vi "Grafici MANAGER REPORT.vi"() -> ()   [LabVIEW 2019]
uses:
  Global percorso impostazioni.vi
  TypeDef/Definizione_plot.ctl
  TypeDef/Definizione_Grafico_REPORT_OLD.ctl
panel:
  out "deleted portion":T1[](array[typedef]) {"PLOT"."GRANDEZZA Y" items=["Banco", "Anno", "Numero", "N° tabella", "Misura", "Tipo prova", "Progressivo Acq", "tempo[h:m:s]", "tempo acq[min]", "f [Hz]", "Uav [V]", "Iav [A]", "Tq [Nm]", "n [rpm]", "P1 [kW]", "P1 n[kW]", "Q [m3/h]", "Q n[m3/h]", "Q [l/min]", "Q n[l/min]", "H1 [m]", "Dislivello [m]", "Hdinamica [m]", "HvAsp [m]", "HvMand [m]", "HvTot [m]", "H2 [m]", "Htot [m]", "Htot n[m]", "P3 (Phyd) [kW]", "P3 (Phyd) n[kW]", "P2 [kW]", "P2 n[kW]", "P2 n ps[kW]", "eta motore [%]", "eta pompa [%]", "eta pompa n[%]", "eta gruppo [%]", "eta gruppo n[%]", "T acqua [°C]", "Densità liquido [kg/m3]", "P barometrica [mbar]", "pf", "Uch1 [V]", "Uch2 [V]", "Uch3 [V]", "Ich1 [A]", "Ich2 [A]", "Ich3 [A]", "Temp.amb[°C]", "Ru-w [ohm]", "DTavvolg. [°C]", "Tamb Freddo [°C]", "Ru-w Freddo [ohm]", "Tc1[°C]", "Tc2[°C]", "Tc3[°C]", "Tc4[°C]", "Tc5", "Tc6", "Tc7", "Tc8", "H1[Bar]", "H2[bar]", "P premist.[Bar]", "Pserb[bar]", "n°NPSH", "NPSH", "Htot Ref[m]", "NPSH_%caduta", "%caduta", "Qref [m3/h]", "MEI"]; "PLOT"."GRANDEZZA X" items=["Banco", "Anno", "Numero", "N° tabella", "Misura", "Tipo prova", "Progressivo Acq", "tempo[h:m:s]", "tempo acq[min]", "f [Hz]", "Uav [V]", "Iav [A]", "Tq [Nm]", "n [rpm]", "P1 [kW]", "P1 n[kW]", "Q [m3/h]", "Q n[m3/h]", "Q [l/min]", "Q n[l/min]", "H1 [m]", "Dislivello [m]", "Hdinamica [m]", "HvAsp [m]", "HvMand [m]", "HvTot [m]", "H2 [m]", "Htot [m]", "Htot n[m]", "P3 (Phyd) [kW]", "P3 (Phyd) n[kW]", "P2 [kW]", "P2 n[kW]", "P2 n ps[kW]", "eta motore [%]", "eta pompa [%]", "eta pompa n[%]", "eta gruppo [%]", "eta gruppo n[%]", "T acqua [°C]", "Densità liquido [kg/m3]", "P barometrica [mbar]", "pf", "Uch1 [V]", "Uch2 [V]", "Uch3 [V]", "Ich1 [A]", "Ich2 [A]", "Ich3 [A]", "Temp.amb[°C]", "Ru-w [ohm]", "DTavvolg. [°C]", "Tamb Freddo [°C]", "Ru-w Freddo [ohm]", "Tc1[°C]", "Tc2[°C]", "Tc3[°C]", "Tc4[°C]", "Tc5", "Tc6", "Tc7", "Tc8", "H1[Bar]", "H2[bar]", "P premist.[Bar]", "Pserb[bar]", "n°NPSH", "NPSH", "Htot Ref[m]", "NPSH_%caduta", "%caduta", "Qref [m3/h]", "MEI"]; "Assi grafico"."ASSE X" items=["X 1", "X 2"]; "Assi grafico"."ASSE Y" items=["Y 1", "Y 2", "Y 3", "Y 4"]}
  out "Array plot":T1[](array[typedef]) {"PLOT"."GRANDEZZA Y" items=["Banco", "Anno", "Numero", "N° tabella", "Misura", "Tipo prova", "Progressivo Acq", "tempo[h:m:s]", "tempo acq[min]", "f [Hz]", "Uav [V]", "Iav [A]", "Tq [Nm]", "n [rpm]", "P1 [kW]", "P1 n[kW]", "Q [m3/h]", "Q n[m3/h]", "Q [l/min]", "Q n[l/min]", "H1 [m]", "Dislivello [m]", "Hdinamica [m]", "HvAsp [m]", "HvMand [m]", "HvTot [m]", "H2 [m]", "Htot [m]", "Htot n[m]", "P3 (Phyd) [kW]", "P3 (Phyd) n[kW]", "P2 [kW]", "P2 n[kW]", "P2 n ps[kW]", "eta motore [%]", "eta pompa [%]", "eta pompa n[%]", "eta gruppo [%]", "eta gruppo n[%]", "T acqua [°C]", "Densità liquido [kg/m3]", "P barometrica [mbar]", "pf", "Uch1 [V]", "Uch2 [V]", "Uch3 [V]", "Ich1 [A]", "Ich2 [A]", "Ich3 [A]", "Temp.amb[°C]", "Ru-w [ohm]", "DTavvolg. [°C]", "Tamb Freddo [°C]", "Ru-w Freddo [ohm]", "Tc1[°C]", "Tc2[°C]", "Tc3[°C]", "Tc4[°C]", "Tc5", "Tc6", "Tc7", "Tc8", "H1[Bar]", "H2[bar]", "P premist.[Bar]", "Pserb[bar]", "n°NPSH", "NPSH", "Htot Ref[m]", "NPSH_%caduta", "%caduta", "Qref [m3/h]", "MEI"]; "PLOT"."GRANDEZZA X" items=["Banco", "Anno", "Numero", "N° tabella", "Misura", "Tipo prova", "Progressivo Acq", "tempo[h:m:s]", "tempo acq[min]", "f [Hz]", "Uav [V]", "Iav [A]", "Tq [Nm]", "n [rpm]", "P1 [kW]", "P1 n[kW]", "Q [m3/h]", "Q n[m3/h]", "Q [l/min]", "Q n[l/min]", "H1 [m]", "Dislivello [m]", "Hdinamica [m]", "HvAsp [m]", "HvMand [m]", "HvTot [m]", "H2 [m]", "Htot [m]", "Htot n[m]", "P3 (Phyd) [kW]", "P3 (Phyd) n[kW]", "P2 [kW]", "P2 n[kW]", "P2 n ps[kW]", "eta motore [%]", "eta pompa [%]", "eta pompa n[%]", "eta gruppo [%]", "eta gruppo n[%]", "T acqua [°C]", "Densità liquido [kg/m3]", "P barometrica [mbar]", "pf", "Uch1 [V]", "Uch2 [V]", "Uch3 [V]", "Ich1 [A]", "Ich2 [A]", "Ich3 [A]", "Temp.amb[°C]", "Ru-w [ohm]", "DTavvolg. [°C]", "Tamb Freddo [°C]", "Ru-w Freddo [ohm]", "Tc1[°C]", "Tc2[°C]", "Tc3[°C]", "Tc4[°C]", "Tc5", "Tc6", "Tc7", "Tc8", "H1[Bar]", "H2[bar]", "P premist.[Bar]", "Pserb[bar]", "n°NPSH", "NPSH", "Htot Ref[m]", "NPSH_%caduta", "%caduta", "Qref [m3/h]", "MEI"]; "Assi grafico"."ASSE X" items=["X 1", "X 2"]; "Assi grafico"."ASSE Y" items=["Y 1", "Y 2", "Y 3", "Y 4"]}
  out "Array grafici":T2[](array[typedef])
  in  "Tab Control":enum32{"GESTIONE GRAFICI", "GESTIONI PLOT"}(tab)
  in  "SALVA plots":bool
  in  "carica plot":bool
  in  "CARICA PLOT GRAFICI":bool
  in  "ELIMINA PLOT":bool
  in  "MODIFICA PLOT":bool
  in  "ELIMINA GRAFICO":bool
  in  "carica grafico":bool
  in  "SALVA GRAFICI":bool
  in  "lista grafici":i32(listbox)
  in  "CREA GRAFICO":bool
  in  "GRAFICO":T2
  in  "exit":bool
  in  "PLOT":T1={"Assi grafico"={"ASSE Y"=0, "ASSE X"=0, "Colore x"=0, "Colore y"=0}, "TIPO COLLEGAMENTO"="", "PLOT"={"GRANDEZZA X"=0, "GRANDEZZA Y"=16, "COLORE PLOT"=0, "NOME PLOT"="", "Larghezza linea"=0, "stile linea"=0, "stile punto"=0}, "NOME GRAFICO"=""} {"PLOT"."GRANDEZZA Y" items=["Banco", "Anno", "Numero", "N° tabella", "Misura", "Tipo prova", "Progressivo Acq", "tempo[h:m:s]", "tempo acq[min]", "f [Hz]", "Uav [V]", "Iav [A]", "Tq [Nm]", "n [rpm]", "P1 [kW]", "P1 n[kW]", "Q [m3/h]", "Q n[m3/h]", "Q [l/min]", "Q n[l/min]", "H1 [m]", "Dislivello [m]", "Hdinamica [m]", "HvAsp [m]", "HvMand [m]", "HvTot [m]", "H2 [m]", "Htot [m]", "Htot n[m]", "P3 (Phyd) [kW]", "P3 (Phyd) n[kW]", "P2 [kW]", "P2 n[kW]", "P2 n ps[kW]", "eta motore [%]", "eta pompa [%]", "eta pompa n[%]", "eta gruppo [%]", "eta gruppo n[%]", "T acqua [°C]", "Densità liquido [kg/m3]", "P barometrica [mbar]", "pf", "Uch1 [V]", "Uch2 [V]", "Uch3 [V]", "Ich1 [A]", "Ich2 [A]", "Ich3 [A]", "Temp.amb[°C]", "Ru-w [ohm]", "DTavvolg. [°C]", "Tamb Freddo [°C]", "Ru-w Freddo [ohm]", "Tc1[°C]", "Tc2[°C]", "Tc3[°C]", "Tc4[°C]", "Tc5", "Tc6", "Tc7", "Tc8", "H1[Bar]", "H2[bar]", "P premist.[Bar]", "Pserb[bar]", "n°NPSH", "NPSH", "Htot Ref[m]", "NPSH_%caduta", "%caduta", "Qref [m3/h]", "MEI"]; "PLOT"."GRANDEZZA X" items=["Banco", "Anno", "Numero", "N° tabella", "Misura", "Tipo prova", "Progressivo Acq", "tempo[h:m:s]", "tempo acq[min]", "f [Hz]", "Uav [V]", "Iav [A]", "Tq [Nm]", "n [rpm]", "P1 [kW]", "P1 n[kW]", "Q [m3/h]", "Q n[m3/h]", "Q [l/min]", "Q n[l/min]", "H1 [m]", "Dislivello [m]", "Hdinamica [m]", "HvAsp [m]", "HvMand [m]", "HvTot [m]", "H2 [m]", "Htot [m]", "Htot n[m]", "P3 (Phyd) [kW]", "P3 (Phyd) n[kW]", "P2 [kW]", "P2 n[kW]", "P2 n ps[kW]", "eta motore [%]", "eta pompa [%]", "eta pompa n[%]", "eta gruppo [%]", "eta gruppo n[%]", "T acqua [°C]", "Densità liquido [kg/m3]", "P barometrica [mbar]", "pf", "Uch1 [V]", "Uch2 [V]", "Uch3 [V]", "Ich1 [A]", "Ich2 [A]", "Ich3 [A]", "Temp.amb[°C]", "Ru-w [ohm]", "DTavvolg. [°C]", "Tamb Freddo [°C]", "Ru-w Freddo [ohm]", "Tc1[°C]", "Tc2[°C]", "Tc3[°C]", "Tc4[°C]", "Tc5", "Tc6", "Tc7", "Tc8", "H1[Bar]", "H2[bar]", "P premist.[Bar]", "Pserb[bar]", "n°NPSH", "NPSH", "Htot Ref[m]", "NPSH_%caduta", "%caduta", "Qref [m3/h]", "MEI"]; "Assi grafico"."ASSE X" items=["X 1", "X 2"]; "Assi grafico"."ASSE Y" items=["Y 1", "Y 2", "Y 3", "Y 4"]}
  in  "lista plot":i32(listbox)
  in  "Add plot":bool
  in  "Y Scale.Visible":bool
  in  "Active Y Scale":i32
  in  "X Scale.Visible":bool
  in  "Active X Scale":i32
  out "CURVE IDRAULICHE QH":cluster{"X":dbl[], "Y":dbl[]}[](graph)
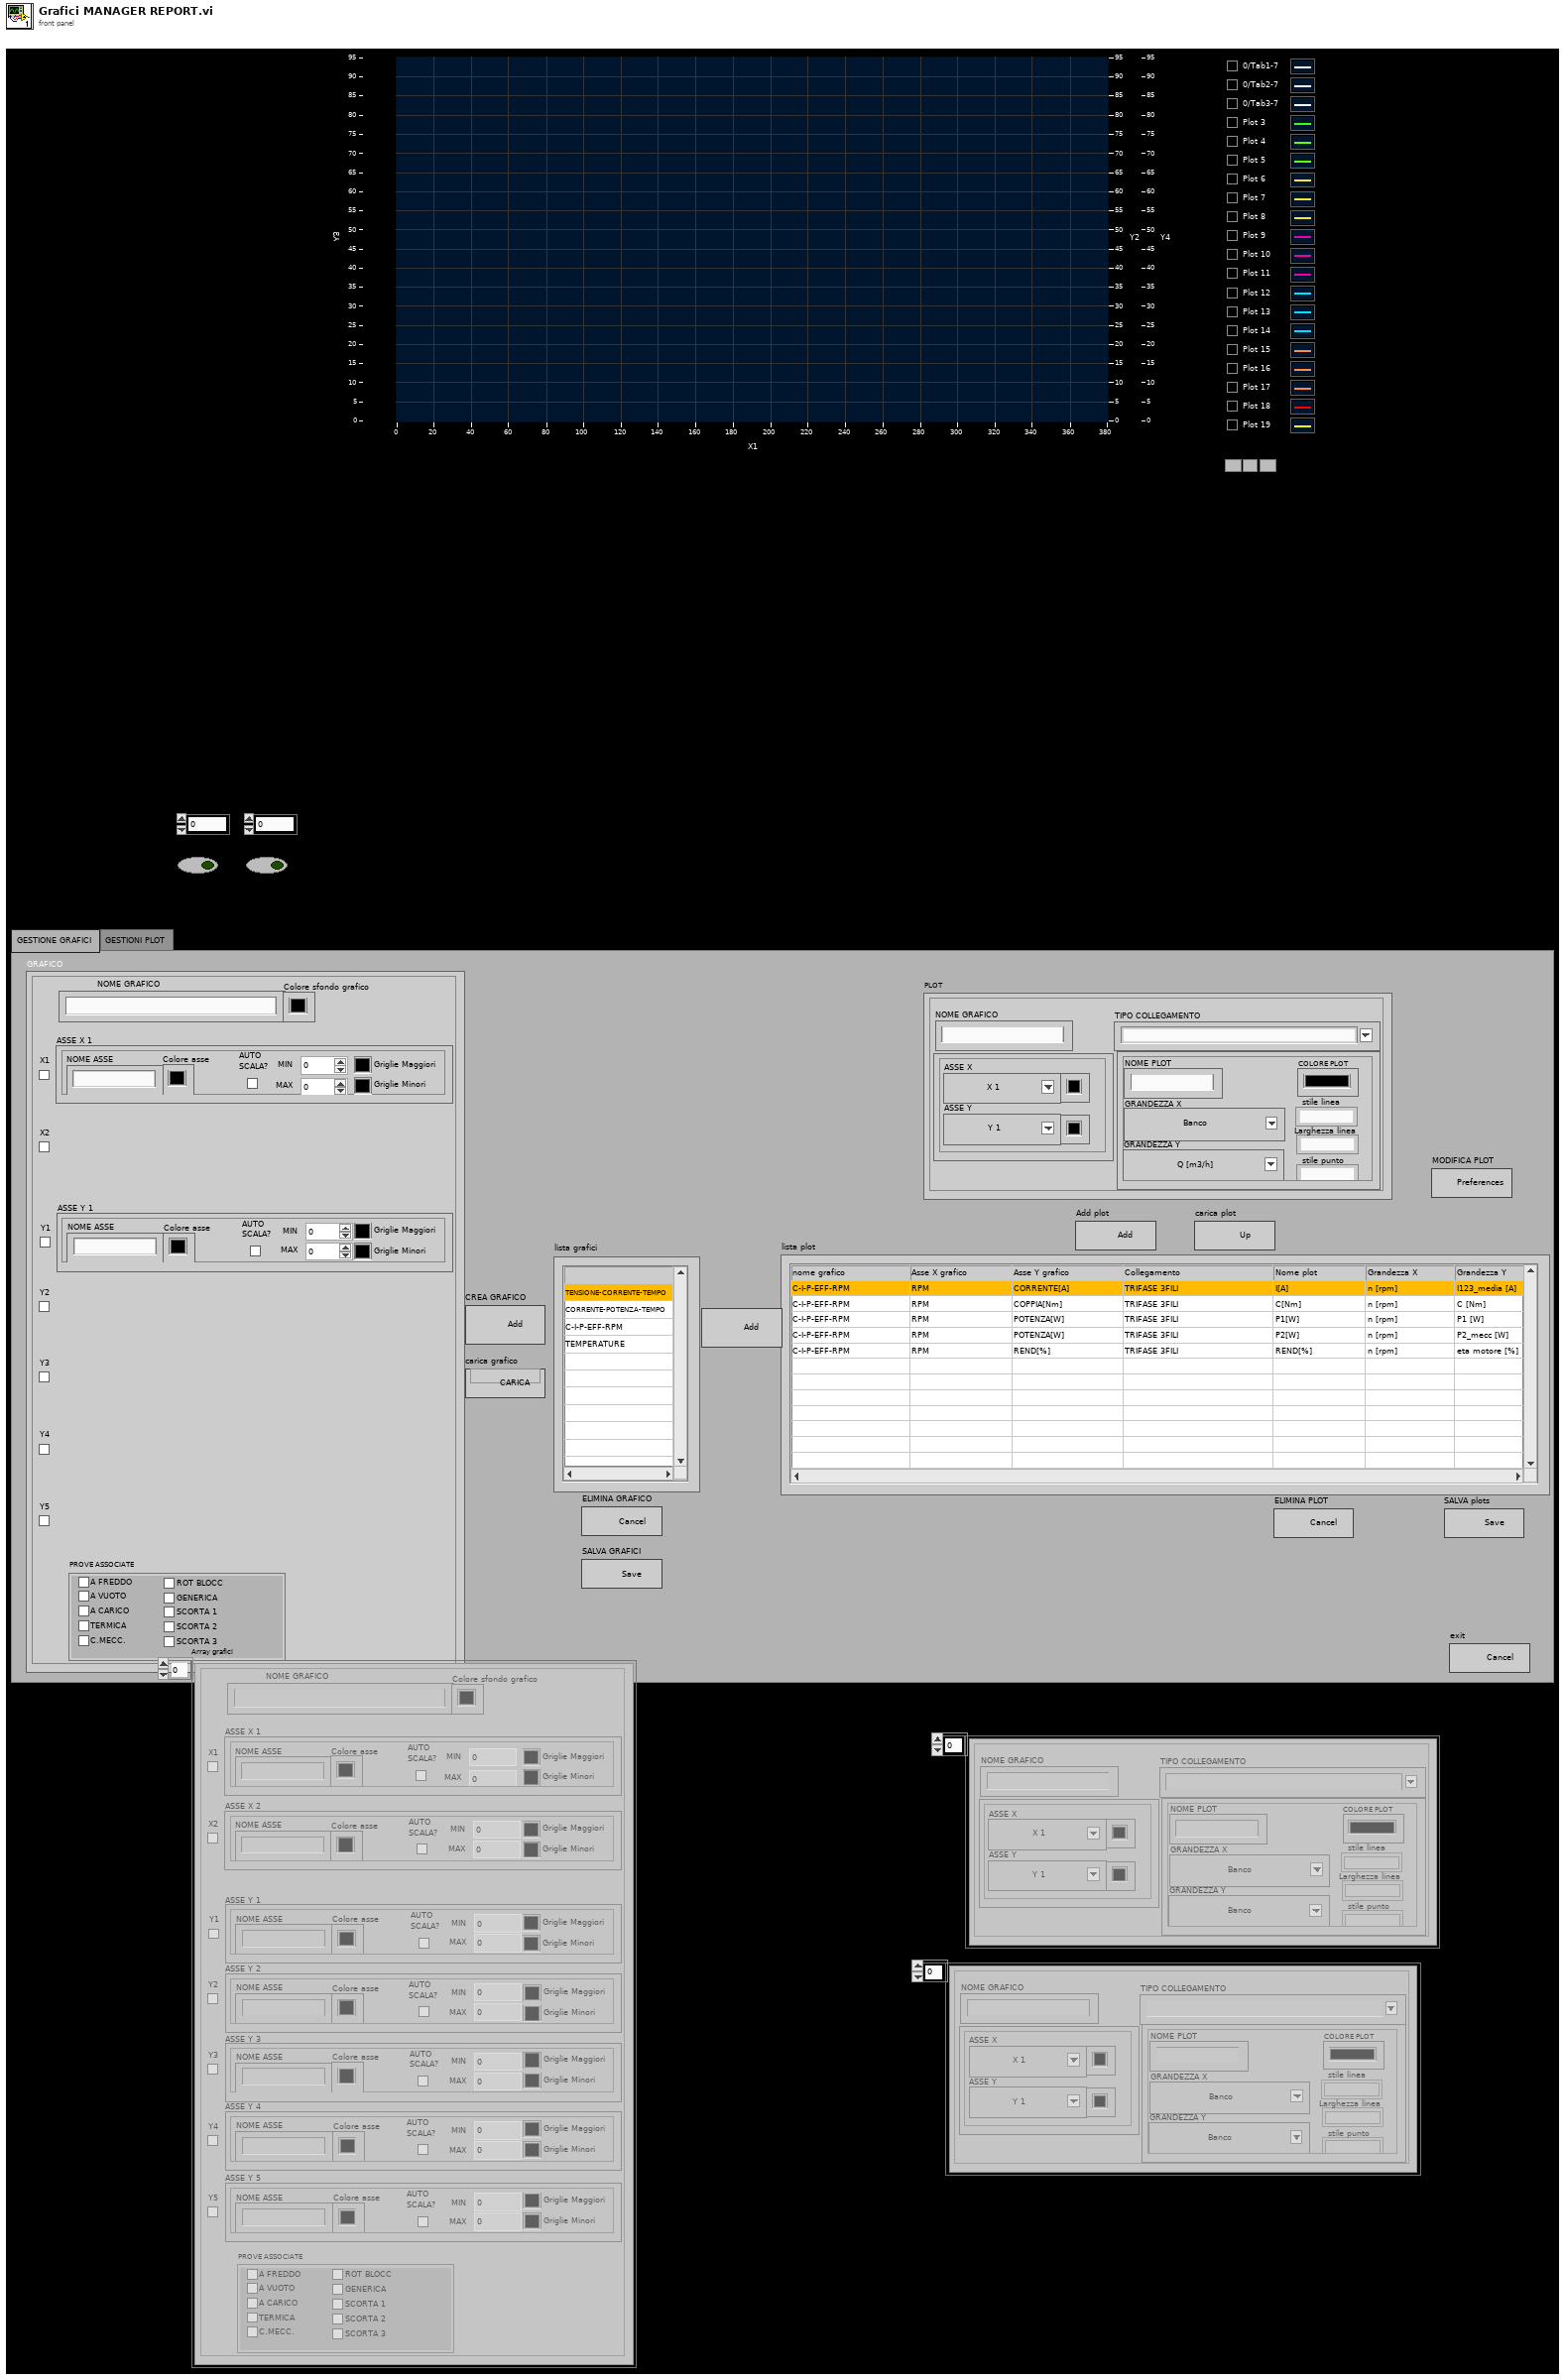
[diagram p1: front panel]
types:
  T1 = typedef "Definizione_plot.ctl" = cluster{"Assi grafico":cluster{"ASSE Y":u16, "ASSE X":u16, "Colore x":u32, "Colore y":u32}, "TIPO COLLEGAMENTO":string, "PLOT":cluster{"GRANDEZZA X":u16, "GRANDEZZA Y":u16, "COLORE PLOT":u32, "NOME PLOT":string, "Larghezza linea":u16, "stile linea":u16, "stile punto":u16}, "NOME GRAFICO":string}
  T2 = typedef "Definizione_Grafico_REPORT_OLD.ctl" = cluster{"ASSE X 1":cluster{"NOME ASSE":string, "AUTO\nSCALA?":bool, "MIN":dbl, "MAX":dbl, "Colore asse":u32, "Griglie Maggiori":u32, "Griglie Minori":u32}, "ASSE X 2":cluster{"NOME ASSE":string, "AUTO\nSCALA?":bool, "MIN":dbl, "MAX":dbl, "Colore asse":u32, "Griglie Maggiori":u32, "Griglie Minori":u32}, "ASSE Y 1":cluster{"NOME ASSE":string, "AUTO\nSCALA?":bool, "MIN":dbl, "MAX":dbl, "Colore asse":u32, "Griglie Maggiori":u32, "Griglie Minori":u32}, "ASSE Y 2":cluster{"NOME ASSE":string, "AUTO\nSCALA?":bool, "MIN":dbl, "MAX":dbl, "Colore asse":u32, "Griglie Maggiori":u32, "Griglie Minori":u32}, "ASSE Y 3":cluster{"NOME ASSE":string, "AUTO\nSCALA?":bool, "MIN":dbl, "MAX":dbl, "Colore asse":u32, "Griglie Maggiori":u32, "Griglie Minori":u32}, "ASSE Y 4":cluster{"NOME ASSE":string, "AUTO\nSCALA?":bool, "MIN":dbl, "MAX":dbl, "Colore asse":u32, "Griglie Maggiori":u32, "Griglie Minori":u32}, "X1":bool, "X2":bool, "Y1":bool, "Y2":bool, "Y3":bool, "Y4":bool, "NOME GRAFICO":string, "PROVE ASSOCIATE":cluster{"A FREDDO":bool, "A VUOTO":bool, "A CARICO":bool, "TERMICA":bool, "C.MECC.":bool, "ROT BLOCC":bool, "GENERICA":bool, "SCORTA 1":bool, "SCORTA 2":bool, "SCORTA 3":bool}, "ASSE Y 5":cluster{"NOME ASSE":string, "AUTO\nSCALA?":bool, "MIN":dbl, "MAX":dbl, "Colore asse":u32, "Griglie Maggiori":u32, "Griglie Minori":u32}, "Y5":bool, "Colore sfondo grafico":u32}
  T3 = enum16{"open", "replace", "create", "open or create", "replace or create", "replace or create with confirmation"}
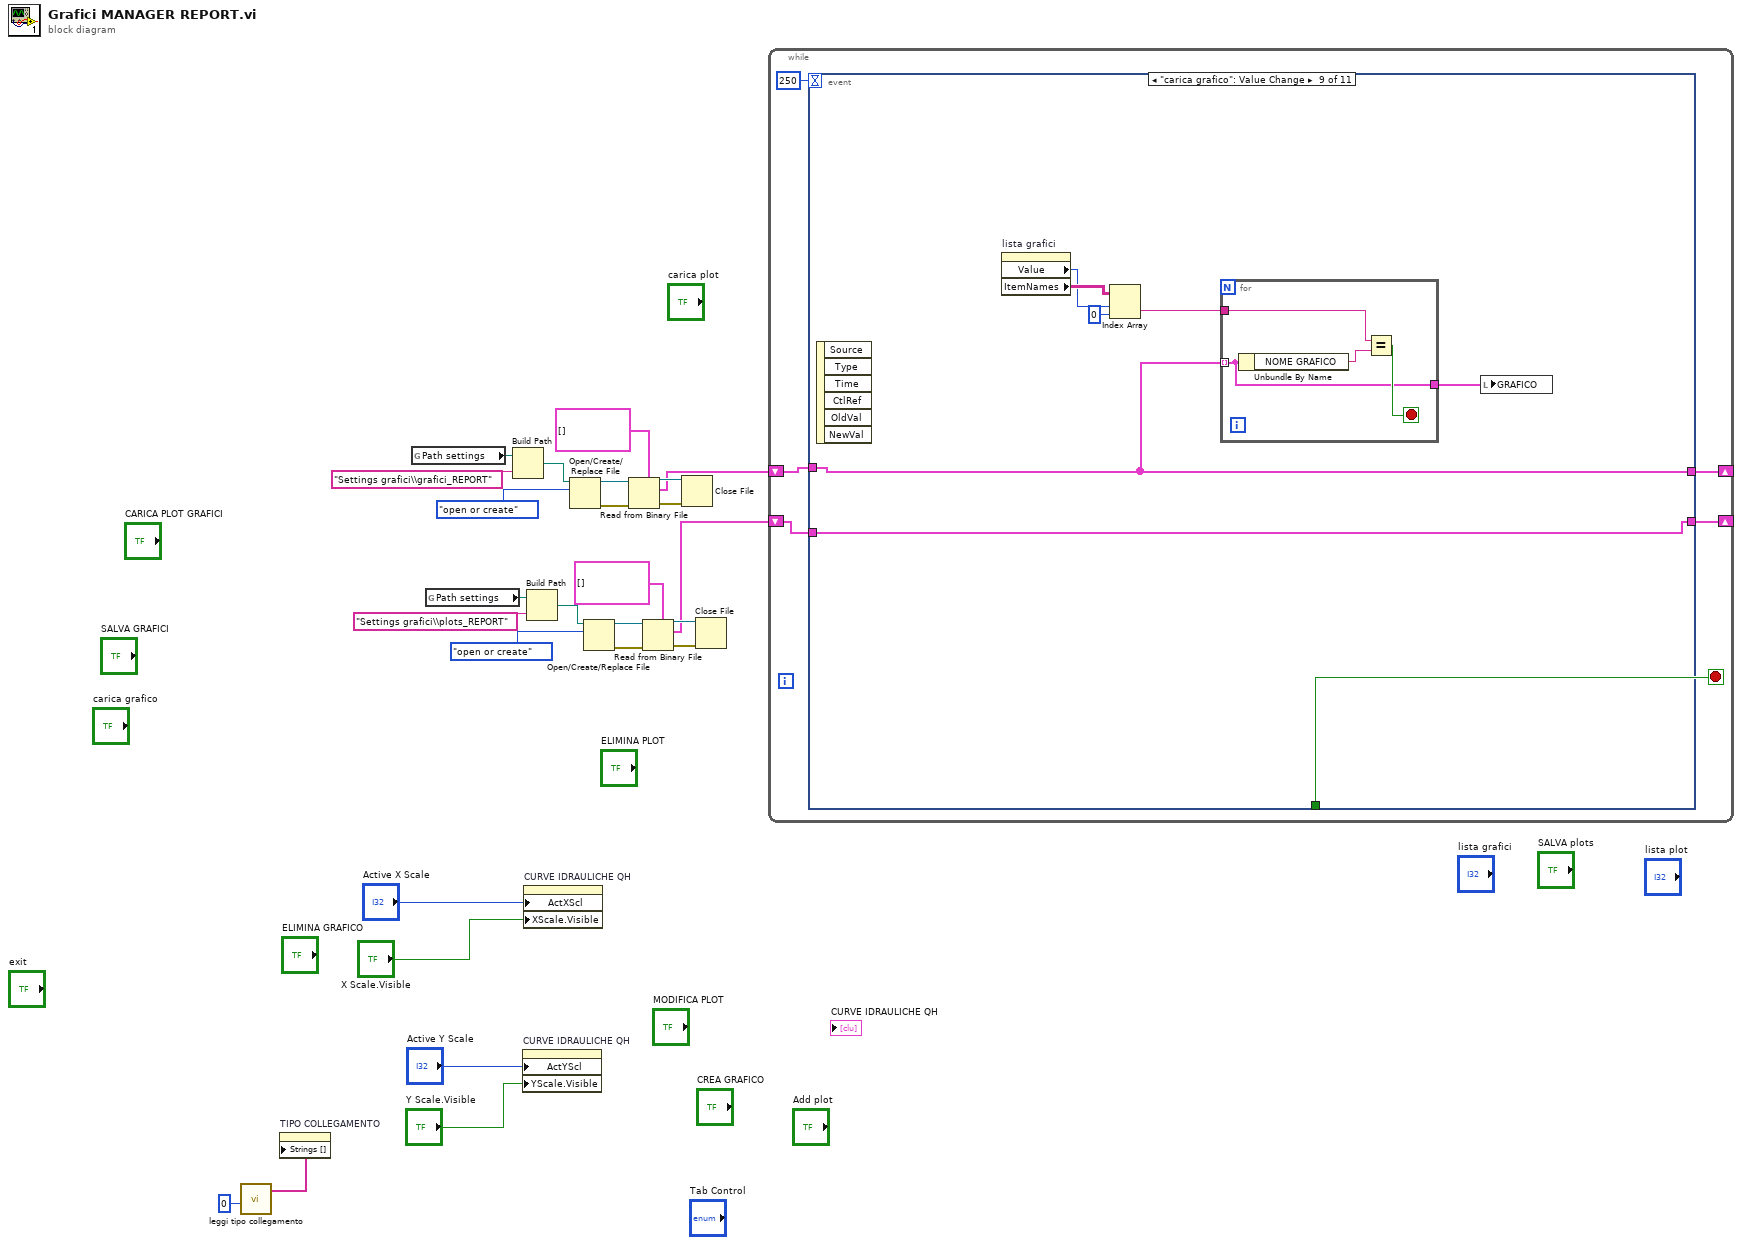
[diagram p0: block diagram]
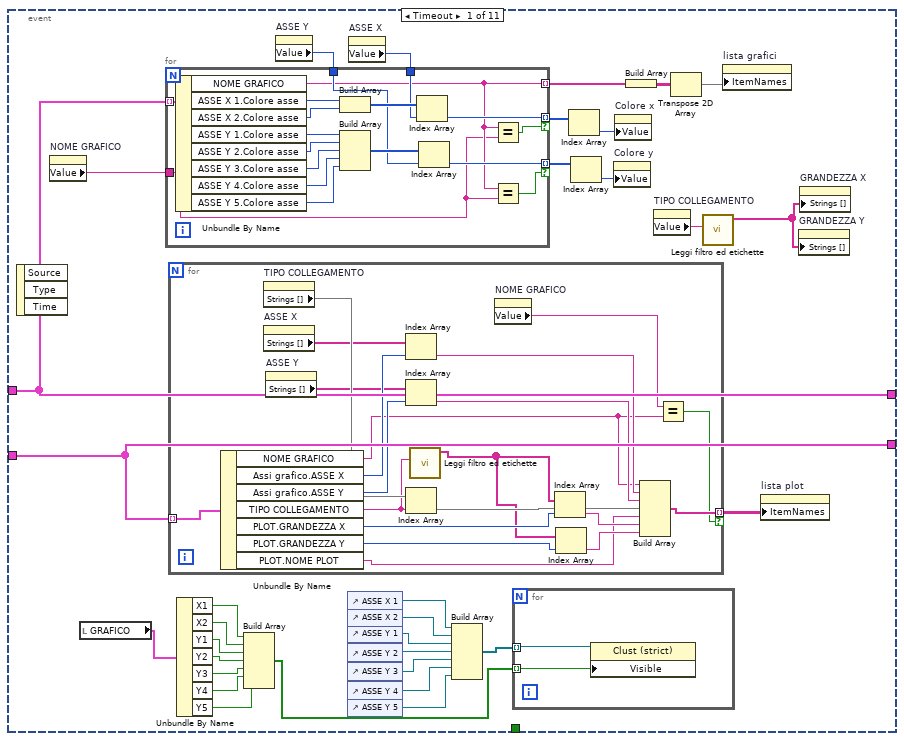
[diagram p2: hidden frame]
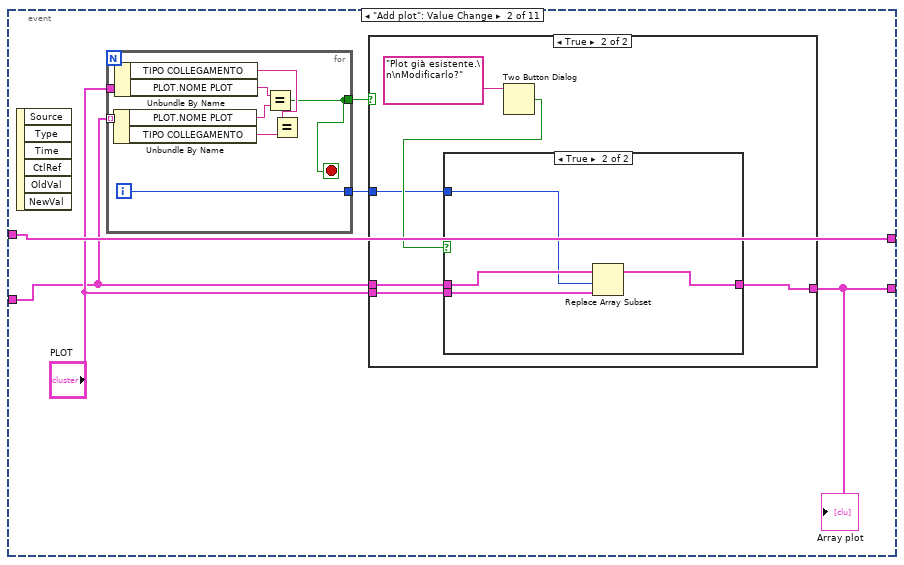
[diagram p3: hidden frame]
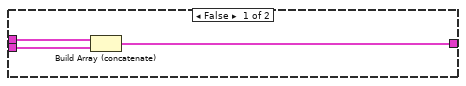
[diagram p4: hidden frame]
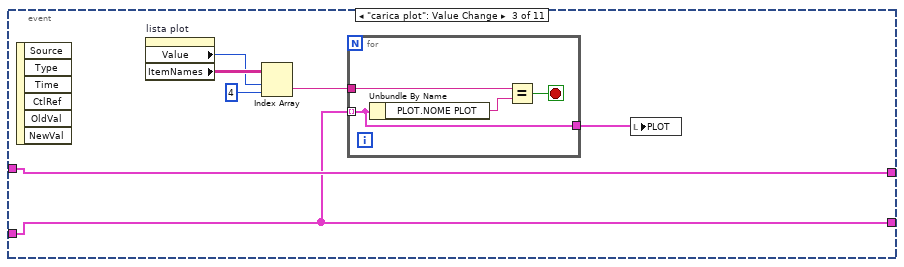
[diagram p6: hidden frame]
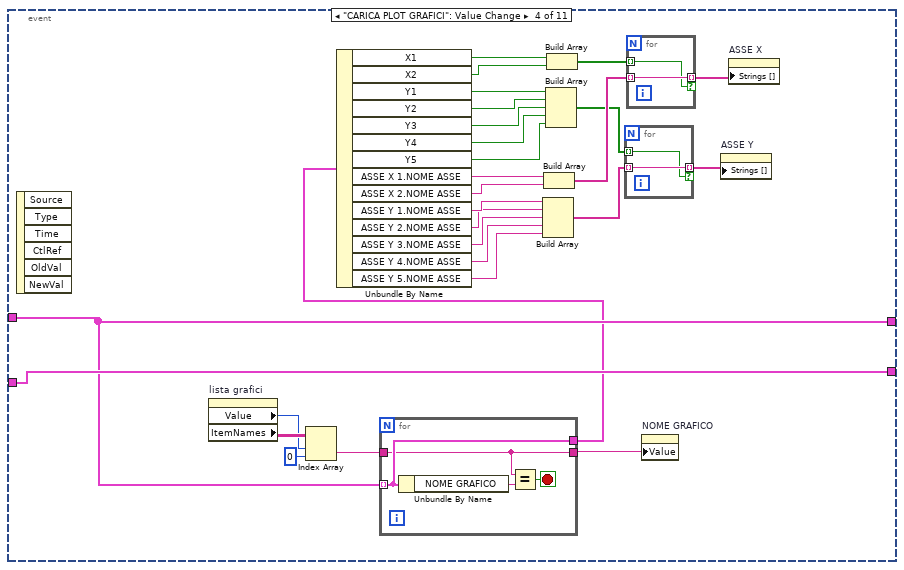
[diagram p7: hidden frame]
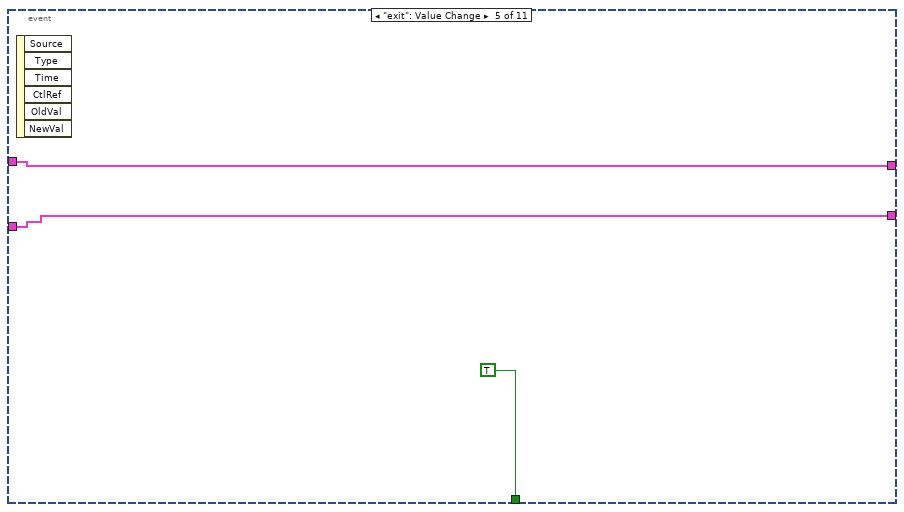
[diagram p8: hidden frame]
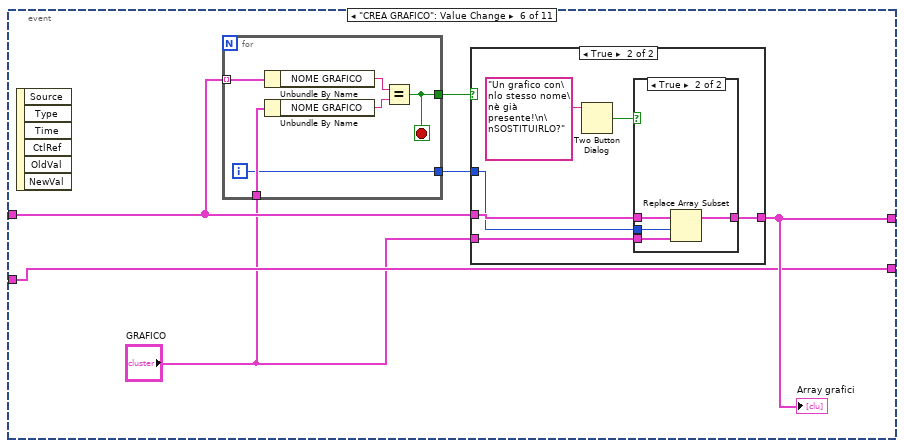
[diagram p9: hidden frame]
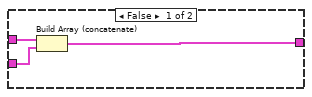
[diagram p10: hidden frame]
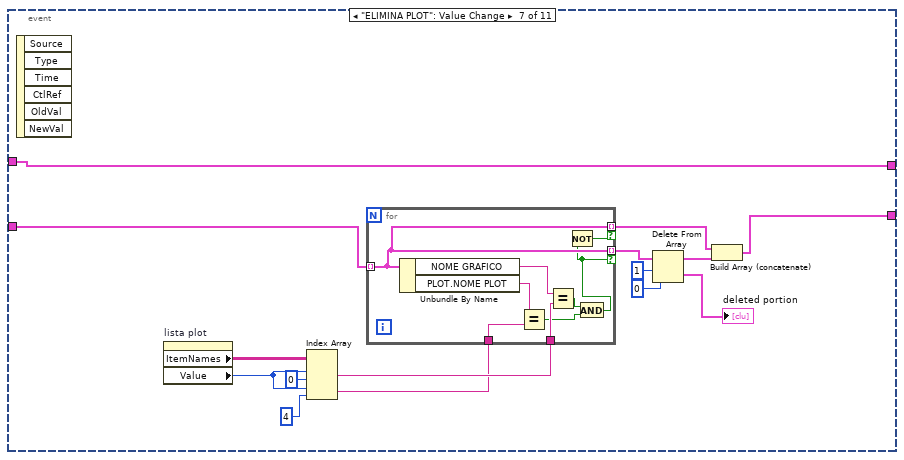
[diagram p12: hidden frame]
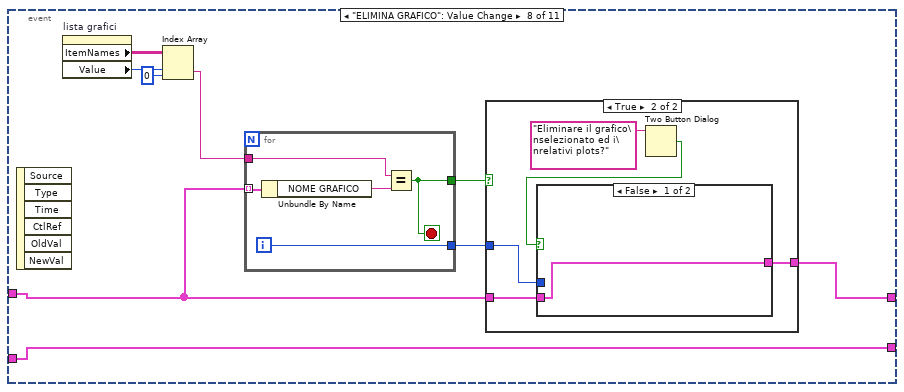
[diagram p13: hidden frame]
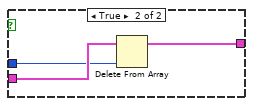
[diagram p15: hidden frame]
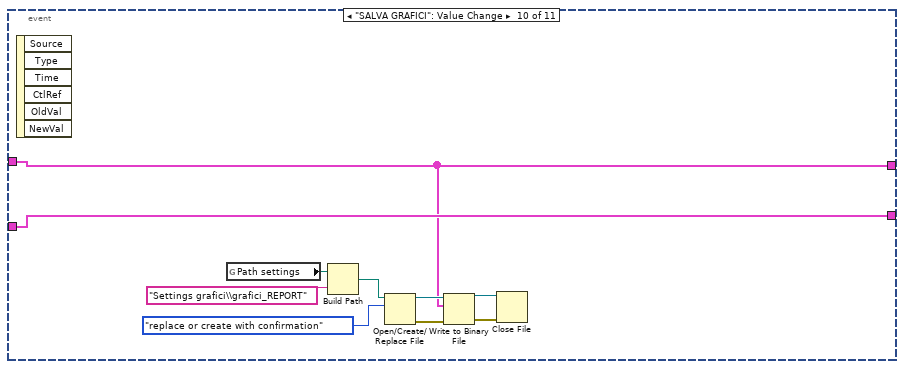
[diagram p16: hidden frame]
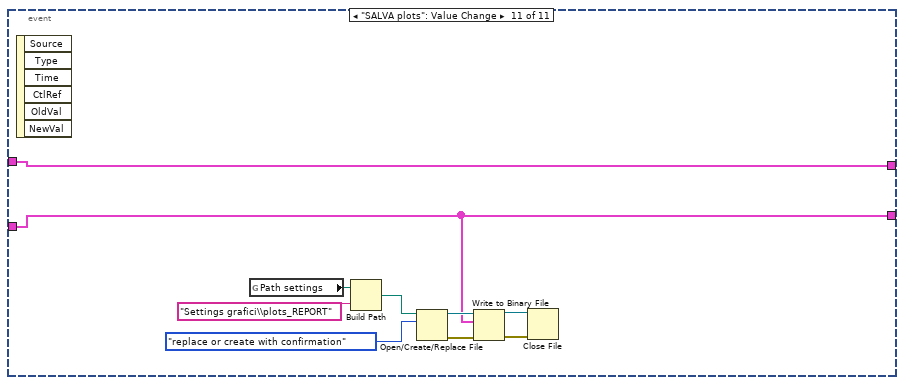
[diagram p17: hidden frame]
diagram:
  n1 = call "leggi tipo collegamento.vi"("lingua"=0) -> ("lista"=w21:string[])  [unwired: 5 in, 5 out]
  n2 = property on="TIPO COLLEGAMENTO" class="CmbBox"("Strings []"=w21) -> ()  [unwired: 2 in, 2 out]
  n3 = global read "Global percorso impostazioni.vi" "Path settings"() -> (w17:path)
  n4 = global read "Global percorso impostazioni.vi" "Path settings"() -> (w6:path)
  n5 = Build Path(base path=w17, name or relative path="Settings grafici\\grafici_REPORT") -> (appended path=w16:path)
  n6 = property on="CURVE IDRAULICHE QH" class="XYGraph (strict)"("ActYScl"="Active Y Scale", "YScale.Visible"="Y Scale.Visible") -> ()  [unwired: 2 in, 2 out]
  n7 = property on="CURVE IDRAULICHE QH" class="XYGraph (strict)"("ActXScl"="Active X Scale", "XScale.Visible"="X Scale.Visible") -> ()  [unwired: 2 in, 2 out]
  n8 = Build Path(base path=w6, name or relative path="Settings grafici\\plots_REPORT") -> (appended path=w7:path)
  n9 = Open/Create/Replace File(file path (use dialog)=w16, operation (0:open)=T3."open or create") -> (refnum out=w14:refnum<file>, error out=w13:errorcluster)  [unwired: 4 in, 1 out]
  n10 = Open/Create/Replace File(file path (use dialog)=w7, operation (0:open)=T3."open or create") -> (refnum out=w9:refnum<file>, error out=w10:errorcluster)  [unwired: 4 in, 1 out]
  n11 = Read from Binary File(5:T2[] [], 8:w13, 11:w14) -> (0:w19:errorcluster, 2:w11:T2[], 3:w20:refnum<file>)  [unwired: 3 in, 1 out]
  n12 = Read from Binary File(5:T1[] [], 8:w10, 11:w9) -> (0:w4:errorcluster, 2:w1:T1[], 3:w3:refnum<file>)  [unwired: 3 in, 1 out]
  n13 = Close File(refnum=w20, error in=w19) -> ()  [unwired: 2 out]
  n14 = Close File(refnum=w3, error in=w4) -> ()  [unwired: 2 out]
  n15 = while {
    shift-right: [w31] -> _
    shift-left: w11 -> [w32]
    shift-right: [w28] -> _
    shift-left: w1 -> [w27]
    stop <- w30 stop-if-true
    n16 = event shown="[8] \"carica grafico\": Value Change" {
      selector: _ -> [_ _ _ _ _ _ _ _ _ _ _]
      dyn-events: _ -> [_ _ _ _ _ _ _ _ _ _ _]
      timeout: 250 -> [_ _ _ _ _ _ _ _ _ _ _]
      tunnel: w32 -> [w64 w109 w139 w166 w181 w186 w223 w235 w259 w270 w287]
      tunnel: [w64 w109 w139 w166 w181 w188 w223 w234 w259 w270 w287] -> w31
      tunnel: [_ _ _ _ TRUE _ _ _ _ _ _] -> w30
      tunnel: [w58 w110 w135 w168 w180 w187 w215 w241 w263 w277 w278] -> w28
      tunnel: w27 -> [w58 w107 w135 w168 w180 w187 w220 w241 w263 w277 w278]
      event Timeout {
        n17 = event-data() -> ()  [unwired: 1 in, 3 out]
        n18 = property on="NOME GRAFICO" class="Str"() -> ("Value"=w39:string)  [unwired: 2 in, 2 out]
        n19 = local read "GRAFICO"() -> (w56:T2)
        n20 = for {
          tunnel: w58 -> [w86] mode=indexing
          tunnel: [w81] -> w57 mode=indexing if=w69
          n21 = Unbundle By Name(w86) -> ("NOME GRAFICO"=w70:string, "Assi grafico.ASSE X"=w79:u16, "Assi grafico.ASSE Y"=w76:u16, "TIPO COLLEGAMENTO"=w68:string, "PLOT.GRANDEZZA X"=w84:u16, "PLOT.GRANDEZZA Y"=w83:u16, "PLOT.NOME PLOT"=w72:string)
          n22 = property on="TIPO COLLEGAMENTO" class="CmbBox"() -> ("Strings []"=w85)  [unwired: 2 in, 2 out]
          n23 = property on="ASSE X" class="Ring (strict)"() -> ("Strings []"=w80:string[])  [unwired: 2 in, 2 out]
          n24 = property on="ASSE Y" class="Ring (strict)"() -> ("Strings []"=w77:string[])  [unwired: 2 in, 2 out]
          n25 = Index Array(array=w80, index=w79) -> (element=w78:string)
          n26 = Index Array(array=w77, index=w76) -> (element=w75:string)
          n27 = Index Array(array=w85, index=w68) -> (element=w82)
          n28 = call "Leggi filtro ed etichette.vi"("ID COLLEGAMENTO"=w68) -> ("ETICHETTE"=w67:string[])  [unwired: 5 in, 5 out]
          n29 = property on="NOME GRAFICO" class="Str"() -> ("Value"=w71:string)  [unwired: 2 in, 2 out]
          n30 = Index Array(array=w67, index=w84) -> (element=w73:string)
          n31 = Index Array(array=w67, index=w83) -> (element=w74:string)
          n32 = Build Array(w70, w78, w75, w82, w72, w73, w74) -> (w81:string[])
          n33 = Equal?(x=w71, y=w70) -> (x = y?=w69:bool)
        }
        n34 = Unbundle By Name(w56) -> ("X1"=w55:bool, "X2"=w54:bool, "Y1"=w53:bool, "Y2"=w52:bool, "Y3"=w51:bool, "Y4"=w50:bool, "Y5"=w41:bool)
        n35 = Build Array(w55, w54, w53, w52, w51, w50, w41) -> (w42:bool[])
        n36 = property on="ASSE Y" class="Ring (strict)"() -> ("Value"=w37:u16)  [unwired: 2 in, 2 out]
        n37 = control-ref of="ASSE X 1"() -> (w49:refnum<vi>)
        n38 = control-ref of="ASSE X 2"() -> (w48:refnum<vi>)
        n39 = control-ref of="ASSE Y 1"() -> (w47:refnum<vi>)
        n40 = control-ref of="ASSE Y 2"() -> (w46:refnum<vi>)
        n41 = control-ref of="ASSE Y 3"() -> (w45:refnum<vi>)
        n42 = control-ref of="ASSE Y 4"() -> (w44:refnum<vi>)
        n43 = control-ref of="ASSE Y 5"() -> (w40:refnum<vi>)
        n44 = property on="ASSE X" class="Ring (strict)"() -> ("Value"=w38:u16)  [unwired: 2 in, 2 out]
        n45 = for {
          tunnel: w64 -> [w104] mode=indexing
          tunnel: [w88] -> w63 mode=indexing
          tunnel: w39 -> [w87]
          tunnel: w38 -> [w94]
          tunnel: w37 -> [w93]
          tunnel: [w92] -> w36 mode=indexing if=w89
          tunnel: [w91] -> w35 mode=indexing if=w90
          n46 = Unbundle By Name(w104) -> ("NOME GRAFICO"=w88:string, "ASSE X 1.Colore asse"=w103:u32, "ASSE X 2.Colore asse"=w102:u32, "ASSE Y 1.Colore asse"=w101:u32, "ASSE Y 2.Colore asse"=w100:u32, "ASSE Y 3.Colore asse"=w99:u32, "ASSE Y 4.Colore asse"=w98:u32, "ASSE Y 5.Colore asse"=w97:u32)
          n47 = Build Array(w103, w102) -> (w96:u32[])
          n48 = Build Array(w101, w100, w99, w98, w97) -> (w95:u32[])
          n49 = Index Array(array=w96, index=w94) -> (element=w92:u32)
          n50 = Index Array(array=w95, index=w93) -> (element=w91:u32)
          n51 = Equal?(x=w88, y=w87) -> (x = y?=w89:bool)
          n52 = Equal?(x=w88, y=w87) -> (x = y?=w90:bool)
        }
        n53 = Build Array(w49, w48, w47, w46, w45, w44, w40) -> (w43:refnum<vi>[])
        n54 = for {
          tunnel: w43 -> [w66] mode=indexing
          tunnel: w42 -> [w65] mode=indexing
          n55 = property class="Clust (strict)"(reference=w66, "Visible"=w65) -> ()  [unwired: 1 in, 2 out]
        }
        n56 = Index Array(array=w36) -> (element=w34:u32)  [unwired: 1 in]
        n57 = Index Array(array=w35) -> (element=w33:u32)  [unwired: 1 in]
        n58 = property on="Colore y" class="ColBox"("Value"=w33) -> ()  [unwired: 2 in, 2 out]
        n59 = property on="Colore x" class="ColBox"("Value"=w34) -> ()  [unwired: 2 in, 2 out]
        n60 = Build Array(w63) -> (w62:string[][])
        n61 = property on="TIPO COLLEGAMENTO" class="CmbBox"() -> ("Value"=w60:string)  [unwired: 2 in, 2 out]
        n62 = Transpose 2D Array(2D array=w62) -> (transposed array=w61:string[][])
        n63 = call "Leggi filtro ed etichette.vi"("ID COLLEGAMENTO"=w60) -> ("ETICHETTE"=w59:string[])  [unwired: 5 in, 5 out]
        n64 = property on="lista grafici" class="MCListbox (strict)"("ItemNames"=w61) -> ()  [unwired: 2 in, 2 out]
        n65 = property on="lista plot" class="MCListbox (strict)"("ItemNames"=w57) -> ()  [unwired: 2 in, 2 out]
        n66 = property on="GRANDEZZA Y" class="Ring (strict)"("Strings []"=w59) -> ()  [unwired: 2 in, 2 out]
        n67 = property on="GRANDEZZA X" class="Ring (strict)"("Strings []"=w59) -> ()  [unwired: 2 in, 2 out]
      }
      event "Add plot": Value Change {
        n68 = event-data() -> ()  [unwired: 1 in, 6 out]
        n69 = for {
          tunnel: "PLOT" -> [w131]
          tunnel: w107 -> [w132] mode=indexing
          tunnel: [w125] -> w106
          tunnel: [w128] -> w105
          i -> [w128]
          stop <- w125 stop-if-true
          n70 = Unbundle By Name(w132) -> ("PLOT.NOME PLOT"=w130:string, "TIPO COLLEGAMENTO"=w127:string)
          n71 = Unbundle By Name(w131) -> ("TIPO COLLEGAMENTO"=w126:string, "PLOT.NOME PLOT"=w129:string)
          n72 = Equal?(x=w129, y=w130) -> (x = y?=w125:bool)
          n73 = Equal?(x=w126, y=w127) -> ()  [unwired: 1 out]
        }
        n74 = case shown="True" w106 {
          tunnel: [w113 w116] -> w110
          tunnel: "PLOT" -> [w112 w114]
          tunnel: w107 -> [w111 w117]
          tunnel: w105 -> [_ w115]
          frame False {
            n75 = Build Array (concatenate)(w111, w112) -> (w113:T1[])
          }
          frame True {
            n76 = Two Button Dialog(message="Plot già esistente.\n\nModificarlo?") -> (T button?=w118:bool)  [unwired: 2 in]
            n77 = case shown="True" w118 {
              tunnel: w117 -> [w120 w124]
              tunnel: [w120 w123] -> w116
              tunnel: w115 -> [_ w122]
              tunnel: w114 -> [_ w121]
              frame False {
              }
              frame True {
                n78 = Replace Array Subset(array=w124, new element=w121, index=w122) -> (w123:T1[])
              }
            }
          }
        }
        "Array plot" <- w110
      }
      event "carica plot": Value Change {
        n79 = event-data() -> ()  [unwired: 1 in, 6 out]
        n80 = property on="lista plot" class="MCListbox (strict)"() -> ("Value"=w136:i32, "ItemNames"=w137:string[][])  [unwired: 2 in, 2 out]
        n81 = Index Array(array=w137, index (row)=w136, index (col)=4 ("disabled index (col)")) -> (element=w134:string)
        n82 = for {
          tunnel: w135 -> [w141] mode=indexing
          tunnel: w134 -> [w142]
          tunnel: [w141] -> w133
          stop <- w140 stop-if-true
          n83 = Unbundle By Name(w141) -> ("PLOT.NOME PLOT"=w143:string)
          n84 = Equal?(x=w142, y=w143) -> (x = y?=w140:bool)
        }
        n85 = local write "PLOT"(w133) -> ()
      }
      event "CARICA PLOT GRAFICI": Value Change {
        n86 = event-data() -> ()  [unwired: 1 in, 6 out]
        n87 = property on="lista grafici" class="MCListbox (strict)"() -> ("Value"=w170:i32, "ItemNames"=w171:string[][])  [unwired: 2 in, 2 out]
        n88 = Index Array(array=w171, index (row)=w170, index (col)=0 ("disabled index (col)")) -> (element=w167:string)
        n89 = for {
          tunnel: w166 -> [w177] mode=indexing
          tunnel: w167 -> [w176]
          tunnel: [w177] -> w147
          tunnel: [w176] -> w146
          stop <- w178 stop-if-true
          n90 = Unbundle By Name(w177) -> ("NOME GRAFICO"=w179:string)
          n91 = Equal?(x=w176, y=w179) -> (x = y?=w178:bool)
        }
        n92 = Unbundle By Name(w147) -> ("X1"=w160:bool, "X2"=w159:bool, "Y1"=w164:bool, "Y2"=w163:bool, "Y3"=w162:bool, "Y4"=w161:bool, "Y5"=w144:bool, "ASSE X 1.NOME ASSE"=w157:string, "ASSE X 2.NOME ASSE"=w156:string, "ASSE Y 1.NOME ASSE"=w155:string, "ASSE Y 2.NOME ASSE"=w154:string, "ASSE Y 3.NOME ASSE"=w153:string, "ASSE Y 4.NOME ASSE"=w165:string, "ASSE Y 5.NOME ASSE"=w145:string)
        n93 = Build Array(w155, w154, w153, w165, w145) -> (w149:string[])
        n94 = Build Array(w157, w156) -> (w152:string[])
        n95 = Build Array(w164, w163, w162, w161, w144) -> (w150:bool[])
        n96 = Build Array(w160, w159) -> (w158:bool[])
        n97 = for {
          tunnel: w150 -> [w172] mode=indexing
          tunnel: w149 -> [w173] mode=indexing
          tunnel: [w173] -> w148 mode=indexing if=w172
        }
        n98 = for {
          tunnel: w158 -> [w174] mode=indexing
          tunnel: w152 -> [w175] mode=indexing
          tunnel: [w175] -> w151 mode=indexing if=w174
        }
        n99 = property on="NOME GRAFICO" class="Str"("Value"=w146) -> ()  [unwired: 2 in, 2 out]
        n100 = property on="ASSE Y" class="Ring (strict)"("Strings []"=w148) -> ()  [unwired: 2 in, 2 out]
        n101 = property on="ASSE X" class="Ring (strict)"("Strings []"=w151) -> ()  [unwired: 2 in, 2 out]
      }
      event "exit": Value Change {
        n102 = event-data() -> ()  [unwired: 1 in, 6 out]
      }
      event "CREA GRAFICO": Value Change {
        n103 = event-data() -> ()  [unwired: 1 in, 6 out]
        n104 = for {
          tunnel: w186 -> [w208] mode=indexing
          tunnel: "GRAFICO" -> [w207]
          tunnel: [w204] -> w185
          tunnel: [w203] -> w184
          i -> [w203]
          stop <- w204 stop-if-true
          n105 = Unbundle By Name(w208) -> ("NOME GRAFICO"=w205:string)
          n106 = Unbundle By Name(w207) -> ("NOME GRAFICO"=w206:string)
          n107 = Equal?(x=w205, y=w206) -> (x = y?=w204:bool)
        }
        n108 = case shown="True" w185 {
          tunnel: [w191 w194] -> w188
          tunnel: w186 -> [w190 w195]
          tunnel: "GRAFICO" -> [w189 w192]
          tunnel: w184 -> [_ w193]
          frame False {
            n109 = Build Array (concatenate)(w190, w189) -> (w191:T2[])
          }
          frame True {
            n110 = Two Button Dialog(message="Un grafico con\nlo stesso nome\nè già presente!\n\nSOSTITUIRLO?") -> (T button?=w196:bool)  [unwired: 2 in]
            n111 = case shown="True" w196 {
              tunnel: w195 -> [w198 w202]
              tunnel: [w198 w199] -> w194
              tunnel: w193 -> [_ w201]
              tunnel: w192 -> [_ w200]
              frame False {
              }
              frame True {
                n112 = Replace Array Subset(array=w202, new element=w200, index=w201) -> (w199:T2[])
              }
            }
          }
        }
        "Array grafici" <- w188
      }
      event "ELIMINA PLOT": Value Change {
        n113 = event-data() -> ()  [unwired: 1 in, 6 out]
        n114 = property on="lista plot" class="MCListbox (strict)"() -> ("ItemNames"=w222:string[][], "Value"=w212:i32)  [unwired: 2 in, 2 out]
        n115 = Index Array(array=w222, index (row) #1=w212, index (col) #1=0 ("disabled index (col)"), index (row) #2=w212, index (col) #2=4 ("disabled index (col)")) -> (element #1=w219:string, element #2=w210:string)
        n116 = for {
          tunnel: w220 -> [w231] mode=indexing
          tunnel: w219 -> [w229]
          tunnel: [w231] -> w218 mode=indexing if=w224
          tunnel: [w231] -> w214 mode=indexing if=w230
          tunnel: w210 -> [w227]
          n117 = Unbundle By Name(w231) -> ("NOME GRAFICO"=w232:string, "PLOT.NOME PLOT"=w228:string)
          n118 = Equal?(x=w228, y=w227) -> (x = y?=w225:bool)
          n119 = Equal?(x=w232, y=w229) -> (x = y?=w226:bool)
          n120 = And(x=w226, y=w225) -> (x .and. y?=w224:bool)
          n121 = Not(x=w224) -> (.not. x?=w230:bool)
        }
        n122 = Delete From Array(array=w218, length=1, index=0) -> (deleted portion=→"deleted portion":T1[], array with subset deleted=w216:T1[])
        n123 = Build Array (concatenate)(w214, w216) -> (w215:T1[])
      }
      event "ELIMINA GRAFICO": Value Change {
        n124 = event-data() -> ()  [unwired: 1 in, 6 out]
        n125 = property on="lista grafici" class="MCListbox (strict)"() -> ("ItemNames"=w240:string[][], "Value"=w239:i32)  [unwired: 2 in, 2 out]
        n126 = Index Array(array=w240, index (row)=w239, index (col)=0 ("disabled index (col)")) -> (element=w237:string)
        n127 = for {
          tunnel: w235 -> [w256] mode=indexing
          tunnel: w237 -> [w254]
          tunnel: [w253] -> w233
          tunnel: [w252] -> w236
          i -> [w253]
          stop <- w252 stop-if-true
          n128 = Unbundle By Name(w256) -> ("NOME GRAFICO"=w255:string)
          n129 = Equal?(x=w254, y=w255) -> (x = y?=w252:bool)
        }
        n130 = case shown="True" w236 {
          tunnel: w235 -> [w242 w246]
          tunnel: [w242 w244] -> w234
          tunnel: w233 -> [_ w243]
          frame False {
          }
          frame True {
            n131 = Two Button Dialog(message="Eliminare il grafico\nselezionato ed i\nrelativi plots?") -> (T button?=w245:bool)  [unwired: 2 in]
            n132 = case shown="False" w245 {
              tunnel: w246 -> [w248 w251]
              tunnel: [w248 w250] -> w244
              tunnel: w243 -> [_ w249]
              frame False {
              }
              frame True {
                n133 = Delete From Array(array=w251, index=w249) -> (array with subset deleted=w250:T2[])  [unwired: 1 in, 1 out]
              }
            }
          }
        }
      }
      event "carica grafico": Value Change {
        n134 = event-data() -> ()  [unwired: 1 in, 6 out]
        n135 = property on="lista grafici" class="MCListbox (strict)"() -> ("Value"=w261:i32, "ItemNames"=w262:string[][])  [unwired: 2 in, 2 out]
        n136 = Index Array(array=w262, index (row)=w261, index (col)=0 ("disabled index (col)")) -> (element=w258:string)
        n137 = for {
          tunnel: w259 -> [w264] mode=indexing
          tunnel: w258 -> [w266]
          tunnel: [w264] -> w257
          stop <- w265 stop-if-true
          n138 = Unbundle By Name(w264) -> ("NOME GRAFICO"=w267:string)
          n139 = Equal?(x=w266, y=w267) -> (x = y?=w265:bool)
        }
        n140 = local write "GRAFICO"(w257) -> ()
      }
      event "SALVA GRAFICI": Value Change {
        n141 = event-data() -> ()  [unwired: 1 in, 6 out]
        n142 = global read "Global percorso impostazioni.vi" "Path settings"() -> (w272:path)
        n143 = Build Path(base path=w272, name or relative path="Settings grafici\\grafici_REPORT") -> (appended path=w273:path)
        n144 = Open/Create/Replace File(file path (use dialog)=w273, operation (0:open)=T3."replace or create with confirmation") -> (refnum out=w275:refnum<file>, error out=w276:errorcluster)  [unwired: 4 in, 1 out]
        n145 = Write to Binary File(file (use dialog)=w275, data=w270, error in=w276) -> (refnum out=w268:refnum<file>, error out=w269:errorcluster)  [unwired: 3 in, 1 out]
        n146 = Close File(refnum=w268, error in=w269) -> ()  [unwired: 2 out]
      }
      event "SALVA plots": Value Change {
        n147 = event-data() -> ()  [unwired: 1 in, 6 out]
        n148 = global read "Global percorso impostazioni.vi" "Path settings"() -> (w282:path)
        n149 = Build Path(base path=w282, name or relative path="Settings grafici\\plots_REPORT") -> (appended path=w283:path)
        n150 = Open/Create/Replace File(file path (use dialog)=w283, operation (0:open)=T3."replace or create with confirmation") -> (refnum out=w285:refnum<file>, error out=w286:errorcluster)  [unwired: 4 in, 1 out]
        n151 = Write to Binary File(file (use dialog)=w285, data=w278, error in=w286) -> (refnum out=w279:refnum<file>, error out=w280:errorcluster)  [unwired: 3 in, 1 out]
        n152 = Close File(refnum=w279, error in=w280) -> ()  [unwired: 2 out]
      }
    }
  }
